vi "CLSUIP_CleanUpAllWires.vi"(8 "error in (no error)":errorcluster, 11 "VI Refnum":refnum<vi>) -> (0 "error out":errorcluster, 3 "VI Refnum out":refnum<vi>)   [LabVIEW 2021, in "MemberVICreation.lvlib"]
uses:
  <resource>/Framework/Providers/LVClassLibrary/NewAccessors/MemberVICreation.lvlib
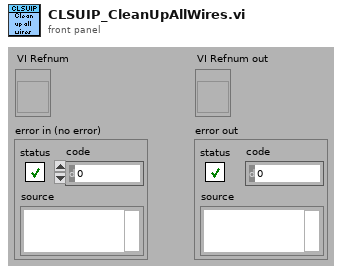
[diagram p1: front panel]
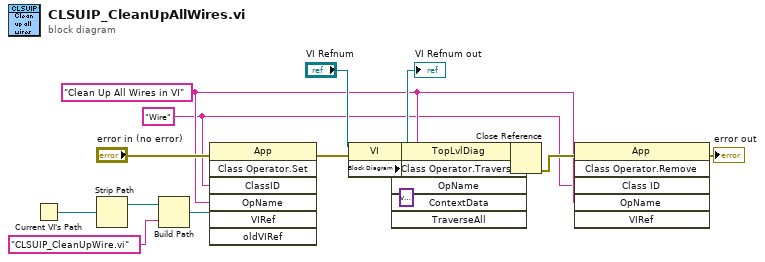
[diagram p0: block diagram]
diagram:
  w5 = "Clean Up All Wires in VI" ("OpName")
  w4 = "Wire" ("ClassName")
  n1 = Current VI's Path() -> (path=w17:path)
  n2 = Strip Path(path=w17) -> (stripped path=w16:path)  [unwired: 1 out]
  n3 = Build Path(base path=w16, name or relative path="CLSUIP_CleanUpWire.vi") -> (appended path=w14:path)
  n4 = invoke class="App" method="Class Operator.Set"(error in="error in (no error)", "ClassID"=w4, "OpName"=w5, "VIRef"=w14) -> (error out=w12:errorcluster)  [unwired: 3 in, 6 out]
  n5 = property class="VI"(reference="VI Refnum", error in=w12) -> (reference out=→"VI Refnum out":refnum<vi>, error out=w11:errorcluster, "Block Diagram"=w3:refnum<vi>)
  n6 = invoke class="TopLvlDiag" method="Class Operator.Traverse"(reference=w3, error in=w11, "OpName"=w5, "ContextData"=variant) -> (reference out=w7:refnum<vi>, error out=w8:errorcluster)  [unwired: 2 in, 4 out]
  n7 = Close Reference(reference=w7, error in (no error)=w8) -> (error out=w6:errorcluster)
  n8 = invoke class="App" method="Class Operator.Remove"(error in=w6, "Class ID"=w4, "OpName"=w5) -> (error out=→"error out":errorcluster)  [unwired: 3 in, 5 out]
